vi "stop.vi"(8 "error in (no error)":errorcluster, 9 "CameraSettings":refnum<class "CamaraSettings.lvclass">, 10 "stop":bool, 11 "Pixelfly in":refnum<class "PixelflySA.lvclass">) -> (0 "error out":errorcluster, 1 "imageSaved":bool, 2 "stopped?":bool, 3 "Pixelfly out":refnum<class "PixelflySA.lvclass">)   [LabVIEW 2009, in "PixelflySA.lvclass"]
uses:
  PixelflySA.lvclass
  Tools/CameraSettings/CamaraSettings.lvclass
  PixelflySA.lvclass/PixelflySA.ctl
  Tools/CameraSettings/PixelFlySettings/PixelflySettings.lvclass
  Channels.lvlib
panel:
  out "Buffer status":T1
  out "Image data":u16[][](graph)
  # "Status flags"
  # "Buffer errors"
  # "Memory usage"
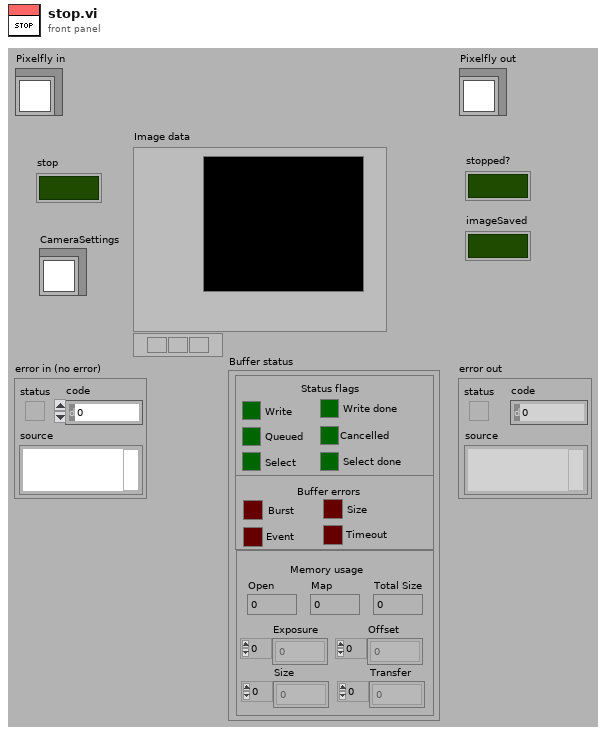
[diagram p1: front panel]
types:
  T1 = cluster{"Write":bool, "Write done":bool, "Queued":bool, "Cancelled":bool, "Select":bool, "Select done":bool, "Burst":bool, "Size":bool, "Event":bool, "Timeout":bool, "Open":i32, "Map":i32, "Exposure":i32[], "Offset":i32[], "Size":i32[], "Transfer":i32[], "Total Size":i32}
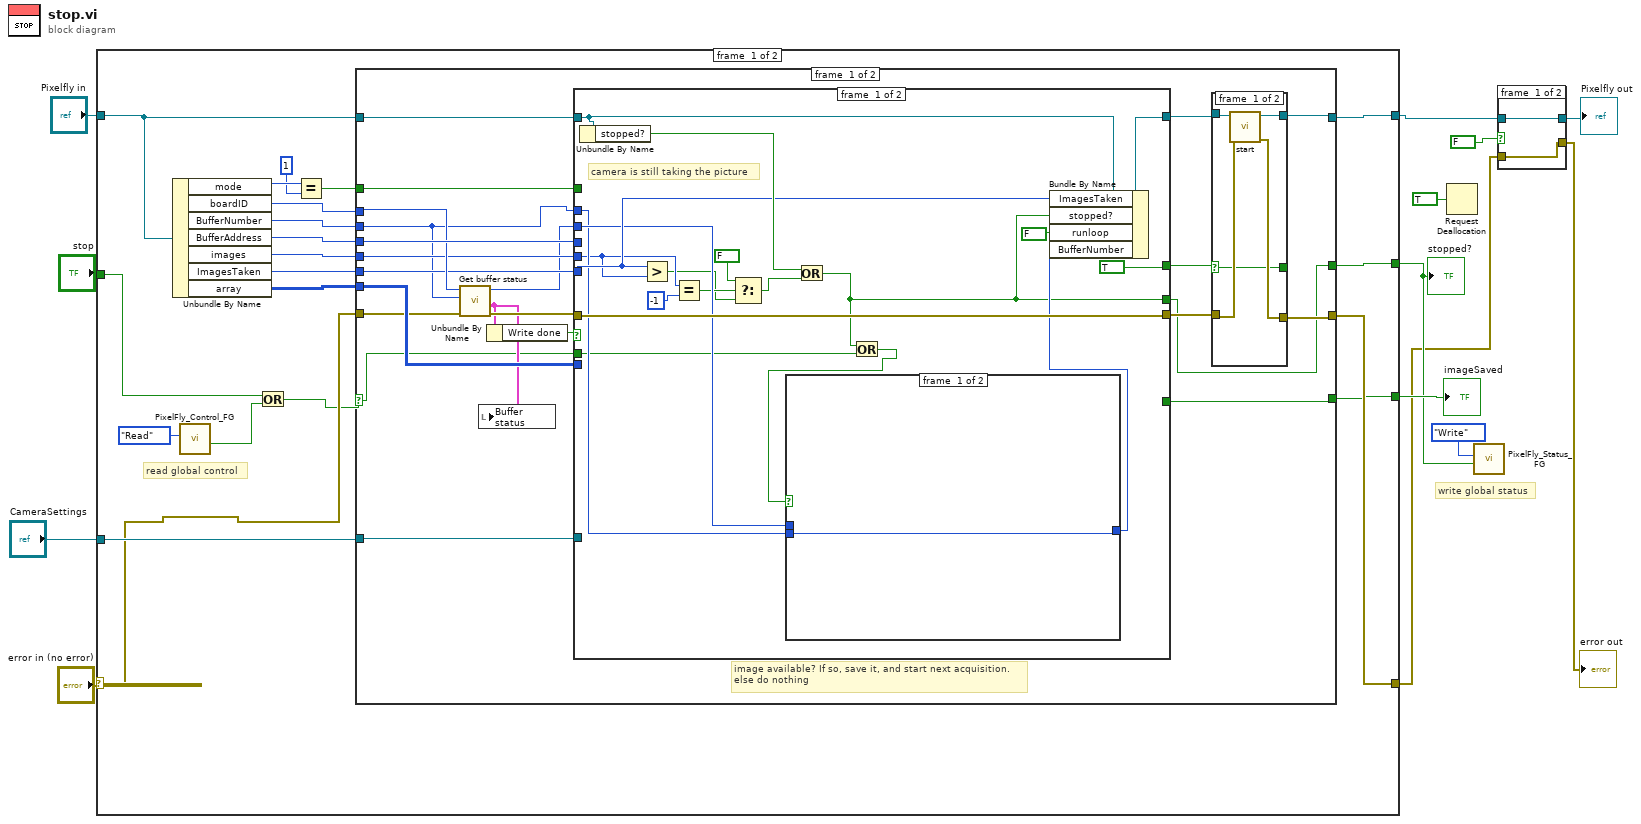
[diagram p0: block diagram]
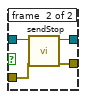
[diagram p2: hidden frame]
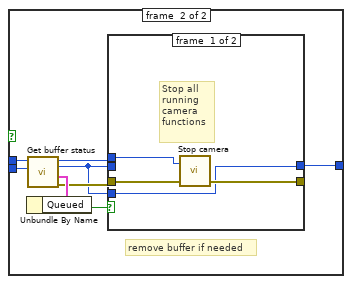
[diagram p4: hidden frame]
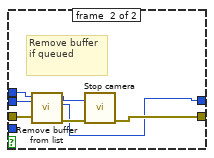
[diagram p5: hidden frame]
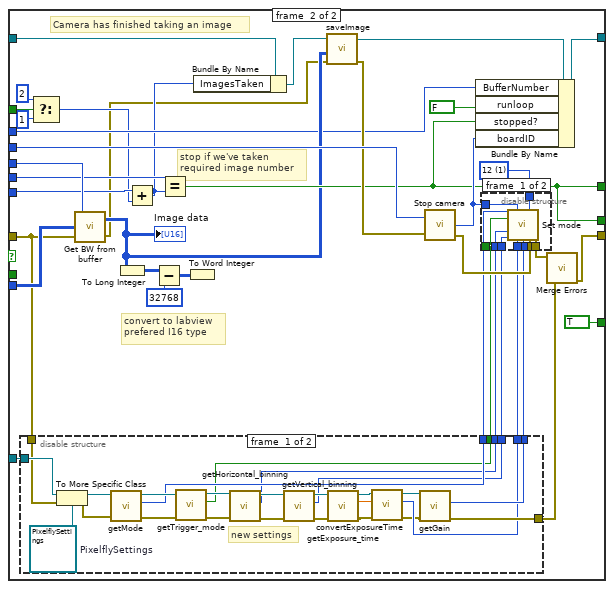
[diagram p6: hidden frame]
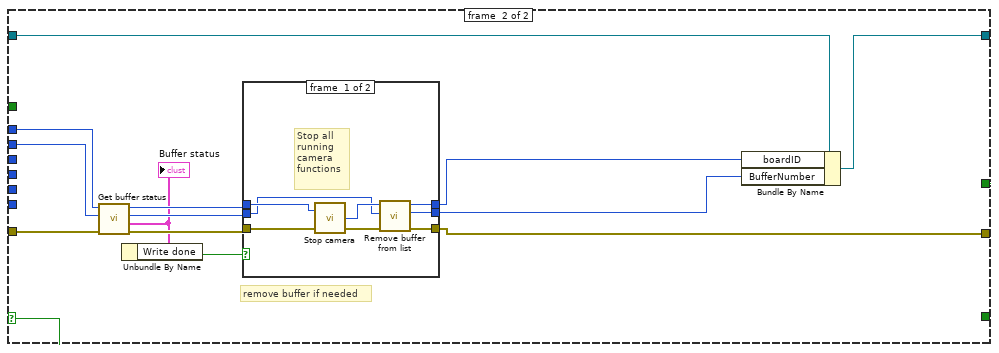
[diagram p9: hidden frame]
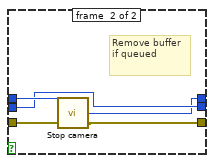
[diagram p10: hidden frame]
diagram:
  # "write global status"
  n1 = case shown="No Error" "error in (no error)" {
    selector: "error in (no error)" -> [w15 w204]
    tunnel: [w30 w204] -> w3
    tunnel: [w29 w205] -> w6
    tunnel: "Pixelfly in" -> [w33 w205]
    tunnel: "stop" -> [w21 _]
    tunnel: [w25 _] -> w4
    tunnel: "CameraSettings" -> [w23 _]
    tunnel: [w22 _] -> w9
    frame #0 {
      # "read global control"
      n2 = Unbundle By Name(w33) -> ("mode"=w18:u16, "boardID"=w32:i32, "BufferNumber"=w31:i32, "BufferAddress"=w26:i32, "images"=w28:i32, "ImagesTaken"=w27:i32, "array"=w24:u16[][])
      n3 = call "PixelFly_Control_FG.vi"("Action"=enum16{"Write", "Read"}."Read") -> ("stopped"=w20:bool)  [unwired: 10 in]
      n4 = Or(x=w21, y=w20) -> (x .or. y?=w14:bool)
      n5 = Equal?(x=w18, y=1) -> (x = y?=w16:bool)
      n6 = case shown="False" w14 {
        selector: w14 -> [w37 w186]
        tunnel: w33 -> [w35 w178]
        tunnel: w32 -> [w53 w190]
        tunnel: w31 -> [w39 w189]
        tunnel: w15 -> [w34 w188]
        tunnel: [w49 w187] -> w30
        tunnel: [w50 w177] -> w29
        tunnel: w28 -> [w45 _]
        tunnel: w27 -> [w47 _]
        tunnel: w26 -> [w54 _]
        tunnel: [w41 w186] -> w25
        tunnel: w24 -> [w48 _]
        tunnel: w23 -> [w43 _]
        tunnel: [w42 _] -> w22
        tunnel: w16 -> [w36 _]
        frame #0 {
          # "image available? If so, save it, and start next acquisition.\nelse do nothing"
          n7 = call <instrlib>:"Get buffer status.vi"("error in (no error)"=w34, "Buffer request"=w39, "Handle in"=w53) -> ("error out"=w40:errorcluster, "Buffer status"=w38:T1, "Handle out"=w44:i32)  [unwired: 1 in, 1 out]
          n8 = local write "Buffer status"(w38) -> ()
          n9 = Unbundle By Name(w38) -> ("Write done"=w55:bool)
          n10 = case shown="True" w55 {
            tunnel: w54 -> [_ w139]
            tunnel: w40 -> [w82 w131]
            tunnel: [w82 w123] -> w51
            tunnel: w47 -> [w77 w110]
            tunnel: w45 -> [w72 w137]
            tunnel: [TRUE w115] -> w52
            tunnel: w48 -> [_ w138]
            tunnel: [w78 w136] -> w46
            tunnel: w35 -> [w79 w105]
            tunnel: w44 -> [w76 w135]
            tunnel: w43 -> [_ w132]
            tunnel: [_ TRUE] -> w42
            tunnel: [w66 w115] -> w41
            tunnel: w39 -> [w75 w112]
            tunnel: w37 -> [w65 _]
            tunnel: w36 -> [_ w109]
            frame #0 {
              # "camera is still taking the picture"
              n11 = Unbundle By Name(w79) -> ("stopped?"=w80:bool)
              n12 = Greater?(x=w77, y=w72) -> (0:w69:bool)
              n13 = Equal?(x=w72, y=-1) -> (x = y?=w71:bool)
              n14 = Select(t=FALSE, s=w71, f=w69) -> (s? t:f=w68:bool)
              n15 = Or(x=w80, y=w68) -> (x .or. y?=w66:bool)
              n16 = Or(x=w66, y=w65) -> (x .or. y?=w64:bool)
              n17 = case shown="True" w64 {
                tunnel: w76 -> [_ w87]
                tunnel: w75 -> [w83 w86]
                tunnel: [w83 w85] -> w67
                frame #0 {
                }
                frame #1 {
                  # "remove buffer if needed"
                  n18 = call <instrlib>:"Get buffer status.vi"("Buffer request"=w86, "Handle in"=w87) -> ("error out"=w90:errorcluster, "Buffer status"=w91:T1, "Buffer number"=w84:i32, "Handle out"=w89:i32)  [unwired: 2 in]
                  n19 = Unbundle By Name(w91) -> ("Queued"=w88:bool)
                  n20 = case shown="True" w88 {
                    tunnel: w90 -> [w94 w96]
                    tunnel: [w93 w101] -> _
                    tunnel: w84 -> [_ w100]
                    tunnel: w89 -> [w95 w97]
                    tunnel: [w92 w99] -> w85
                    tunnel: w84 -> [w92 _]
                    frame #0 {
                      # "Stop all running camera functions"
                      n21 = call <instrlib>:"Stop camera.vi"("Handle in"=w95, "error in (no error)"=w94) -> ("error out"=w93:errorcluster)  [unwired: 2 out]
                    }
                    frame #1 {
                      # "Remove buffer if queued"
                      n22 = call <instrlib>:"Remove buffer from list.vi"("error in (no error)"=w96, "Buffer in"=w100, "Handle in"=w97) -> ("error out"=w101:errorcluster, "Buffer number"=w99:i32, "Handle out"=w98:i32)  [unwired: 2 in]
                      n23 = call <instrlib>:"Stop camera.vi"("Handle in"=w98) -> ()  [unwired: 1 in, 3 out]
                    }
                  }
                }
              }
              n24 = Bundle By Name(cluster=w79, "ImagesTaken"=w77, "stopped?"=w66, "runloop"=FALSE, "BufferNumber"=w67) -> (w78:refnum<class "PixelflySA.lvclass">)
            }
            frame #1 {
              w129 = 1 items=["8", "12"] ("bits/pixel")
              # "stop if we've taken \nrequired image number"
              # "Camera has finished taking an image"
              # "convert to labview \nprefered I16 type"
              n25 = disable-structure shown="Enabled" {
                disable-tunnel: w132 -> [w156 _]
                disable-tunnel: w131 -> [w155 w165]
                disable-tunnel: [w151 _] -> w130
                disable-tunnel: [w150 _] -> w128
                disable-tunnel: [w149 _] -> w127
                disable-tunnel: [w148 _] -> w126
                disable-tunnel: [w147 _] -> w125
                disable-tunnel: [w146 w165] -> w122
                disable-tunnel: [w143 _] -> w120
                frame #0 {
                  w157 = refnum<class "PixelflySettings.lvclass"> refnum  # PixelflySettings
                  # "new settings"
                  n26 = To More Specific Class(target class=w157, reference=w156, error in=w155) -> (specific class reference=w154:refnum<class "PixelflySettings.lvclass">, error out=w153:errorcluster)
                  n27 = call "getMode.vi"("error in (no error)"=w153, "PixelflySettings in"=w154) -> ("error out"=w159:errorcluster, "mode"=w151:u16, "PixelflySettings out"=w158:refnum<class "PixelflySettings.lvclass">)  [unwired: 7 in]
                  n28 = call "getTrigger_mode.vi"("error in (no error)"=w159, "PixelflySettings in"=w158) -> ("error out"=w152:errorcluster, "trigger_mode"=w150:bool, "PixelflySettings out"=w160:refnum<class "PixelflySettings.lvclass">)  [unwired: 7 in]
                  n29 = call "getHorizontal_binning.vi"("error in (no error)"=w152, "PixelflySettings in"=w160) -> ("error out"=w162:errorcluster, "horizontal_binning"=w149:enum16{"1", "2"}, "PixelflySettings out"=w161:refnum<class "PixelflySettings.lvclass">)  [unwired: 7 in]
                  n30 = call "getVertical_binning.vi"("error in (no error)"=w162, "PixelflySettings in"=w161) -> ("error out"=w164:errorcluster, "vertical_binning"=w148:enum16{"1", "2"}, "PixelflySettings out"=w163:refnum<class "PixelflySettings.lvclass">)  [unwired: 7 in]
                  n31 = call "getExposure_time.vi"("error in (no error)"=w164, "PixelflySettings in"=w163) -> ("error out"=w142:errorcluster, "exposure_time"=w140:dbl, "PixelflySettings out"=w145:refnum<class "PixelflySettings.lvclass">)  [unwired: 7 in]
                  n32 = call "convertExposureTime.vi"("error in (no error)"=w142, "time s"=w140, "PixelflySettings in"=w145) -> ("error out"=w141:errorcluster, "exposureTime"=w143:i32, "PixelflySettings out"=w144:refnum<class "PixelflySettings.lvclass">)  [unwired: 6 in]
                  n33 = call "getGain.vi"("error in (no error)"=w141, "PixelflySettings in"=w144) -> ("error out"=w146:errorcluster, "gain"=w147:enum16{"Low", "High"})  [unwired: 7 in, 1 out]
                }
                frame #1 {
                }
              }
              n34 = Select(t=2, s=w109, f=1) -> (s? t:f=w106:i32)
              n35 = call <instrlib>:"Get BW from buffer.vi"("error in (no error)"=w131, "Array input"=w138, "Buffer address"=w139) -> ("error out"=w102:errorcluster, "Image data"=w114:u16[][])
              "Image data" <- w114
              n36 = To Long Integer(number=w114) -> (32bit integer=w117:i32[][])
              n37 = Add(x=w110, y=w106) -> (x+y=w103:i32)
              n38 = Subtract(x=w117, y=32768) -> (x-y=w118:i32[][])
              n39 = Equal?(x=w137, y=w103) -> (x = y?=w115:bool)
              n40 = To Word Integer(number=w118) -> ()  [unwired: 1 out]
              n41 = Bundle By Name(cluster=w105, "ImagesTaken"=w103) -> (w104:refnum<class "PixelflySA.lvclass">)
              n42 = call "saveImage.vi"("error in (no error)"=w102, "I16bit image data"=w114, "Pixelfly in"=w104) -> ("error out"=w119:errorcluster, "Pixelfly out"=w111:refnum<class "PixelflySA.lvclass">)  [unwired: 7 in]
              n43 = call <instrlib>:"Stop camera.vi"("Handle in"=w135, "error in (no error)"=w119) -> ("Handle out"=w134:i32, "error out"=w133:errorcluster)  [unwired: 1 out]
              n44 = Bundle By Name(cluster=w111, "BufferNumber"=w112, "runloop"=FALSE, "stopped?"=w115, "boardID"=w134) -> (w136:refnum<class "PixelflySA.lvclass">)
              n45 = disable-structure shown="Enabled" {
                disable-tunnel: w134 -> [w175 _]
                disable-tunnel: w133 -> [w174 w176]
                disable-tunnel: w130 -> [w173 _]
                disable-tunnel: w129 -> [w172 _]
                disable-tunnel: w128 -> [w171 _]
                disable-tunnel: w127 -> [w170 _]
                disable-tunnel: w126 -> [w169 _]
                disable-tunnel: w125 -> [w168 _]
                disable-tunnel: [w167 w176] -> w124
                disable-tunnel: w120 -> [w166 _]
                frame #0 {
                  n46 = call <instrlib>:"Set mode.vi"("Exposure mode"=w173, "Handle in"=w175, "bits/pixel"=w172, "trigger"=w171, "H bin"=w170, "V bin"=w169, "exp time"=w166, "gain"=w168, "error in (no error)"=w174) -> ("error out"=w167:errorcluster)  [unwired: 6 in]
                }
                frame #1 {
                }
              }
              n47 = call <vilib>:"Merge Errors.vi"("error in 2 (no error)"=w122, "error in 1 (no error)"=w124) -> ("error out"=w123:errorcluster)  [unwired: 5 in]
            }
          }
          n48 = case shown="False" w52 {
            selector: w52 -> [w57 w62]
            tunnel: w51 -> [w59 w63]
            tunnel: [w60 w61] -> w50
            tunnel: [w58 w63] -> w49
            tunnel: [w57 w62] -> _
            tunnel: w46 -> [w56 w61]
            frame #0 {
              n49 = call "start.vi"("error in (no error)"=w59, "Pixelfly in"=w56) -> ("error out"=w58:errorcluster, "Pixelfly out"=w60:refnum<class "PixelflySA.lvclass">)  [unwired: 8 in]
            }
            frame #1 {
            }
          }
        }
        frame #1 {
          # "remove buffer if needed"
          n50 = call <instrlib>:"Get buffer status.vi"("error in (no error)"=w188, "Buffer request"=w189, "Handle in"=w190) -> ("error out"=w185:errorcluster, "Buffer status"=w181:T1, "Buffer number"=w184:i32, "Handle out"=w183:i32)  [unwired: 1 in]
          "Buffer status" <- w181
          n51 = Unbundle By Name(w181) -> ("Write done"=w182:bool)
          n52 = case shown="True" w182 {
            tunnel: w185 -> [w197 w203]
            tunnel: [w195 w201] -> w187
            tunnel: w184 -> [w193 w200]
            tunnel: w183 -> [w198 w202]
            tunnel: [w192 w200] -> w179
            tunnel: [w191 w199] -> w180
            frame #0 {
              # "Stop all running camera functions"
              n53 = call <instrlib>:"Stop camera.vi"("Handle in"=w198, "error in (no error)"=w197) -> ("Handle out"=w194:i32, "error out"=w196:errorcluster)  [unwired: 1 out]
              n54 = call <instrlib>:"Remove buffer from list.vi"("error in (no error)"=w196, "Buffer in"=w193, "Handle in"=w194) -> ("error out"=w195:errorcluster, "Buffer number"=w192:i32, "Handle out"=w191:i32)  [unwired: 2 in]
            }
            frame #1 {
              # "Remove buffer if queued"
              n55 = call <instrlib>:"Stop camera.vi"("Handle in"=w202, "error in (no error)"=w203) -> ("Handle out"=w199:i32, "error out"=w201:errorcluster)  [unwired: 1 out]
            }
          }
          n56 = Bundle By Name(cluster=w178, "boardID"=w180, "BufferNumber"=w179) -> (w177:refnum<class "PixelflySA.lvclass">)
        }
      }
    }
    frame #1 {
    }
  }
  "stopped?" <- w4
  "imageSaved" <- w9
  n57 = Request Deallocation(TRUE ("flag")) -> ()
  n58 = call "PixelFly_Status_FG.vi"("stop"=w4, "Action"=enum16{"Write", "Read"}."Write") -> ()  [unwired: 9 in, 1 out]
  n59 = case shown="True" FALSE {
    tunnel: w6 -> [w207 w211]
    tunnel: [w207 w210] -> w5
    tunnel: w3 -> [w206 w209]
    tunnel: [w206 w208] -> w2
    frame #0 {
    }
    frame #1 {
      n60 = call "sendStop.vi"("error in (no error)"=w209, "PixelflySA in"=w211) -> ("error out"=w208:errorcluster, "PixelflySA out"=w210:refnum<class "PixelflySA.lvclass">)  [unwired: 8 in]
    }
  }
  "error out" <- w2
  "Pixelfly out" <- w5
